vi "MeasLeakRate_20.vi"() -> ()   [LabVIEW 2011]
panel:
  out "angle (°)":dbl
  out "Status":string
  out "error out":errorcluster
  out "fit":cluster{"element":dbl, "Value":dbl}[](array[cluster])
  out "T-T0,P":cluster{"element":dbl, "element":dbl}[](array[cluster])
  out "t0":dbl format="%#_8f"
  out "XY Graph":T1(graph)
  out "S00":i32
  out "S20":dbl
  out "S11":dbl
  out "S10":dbl
  out "S01":dbl
  out "T,P":cluster{"element":dbl, "element":dbl}[](array[cluster])
  out "dPdt":dbl
  out "P0":dbl
  out "average P (Torr)":string
  in  "Control Valve Local":bool
  in  "Exhaust Close":bool
  in  "Exhaust Open":bool
  in  "Control Close":bool
  in  "Control Open":bool
  in  "reset":bool
  in  "# points to watch":i32=60
  out "leak rate (torr/min)":string
  out "P":dbl
  out "first":bool=TRUE
  in  "interval (s)":dbl=0.5
  in  "stop":bool
  out "P(torr)":string
  # "Pressure control valve:"
  # "Exahaust valve:"
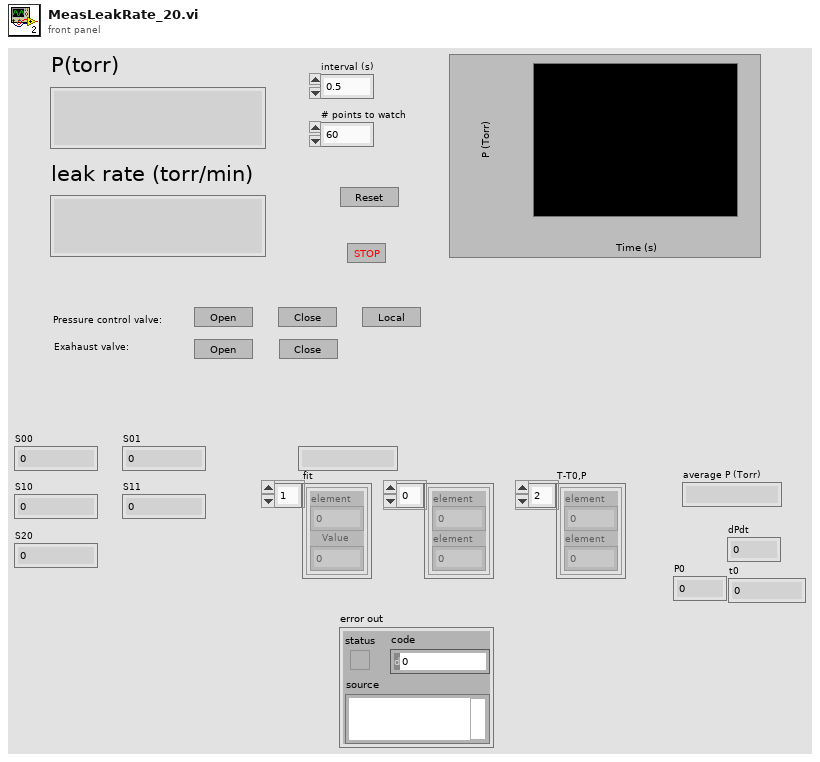
[diagram p1: front panel]
types:
  T1 = cluster{"Value":cluster{"element":dbl, "element":dbl}[]}[]
  T2 = cluster{"Value":cluster{"element":dbl, "Value":dbl}[]}[]
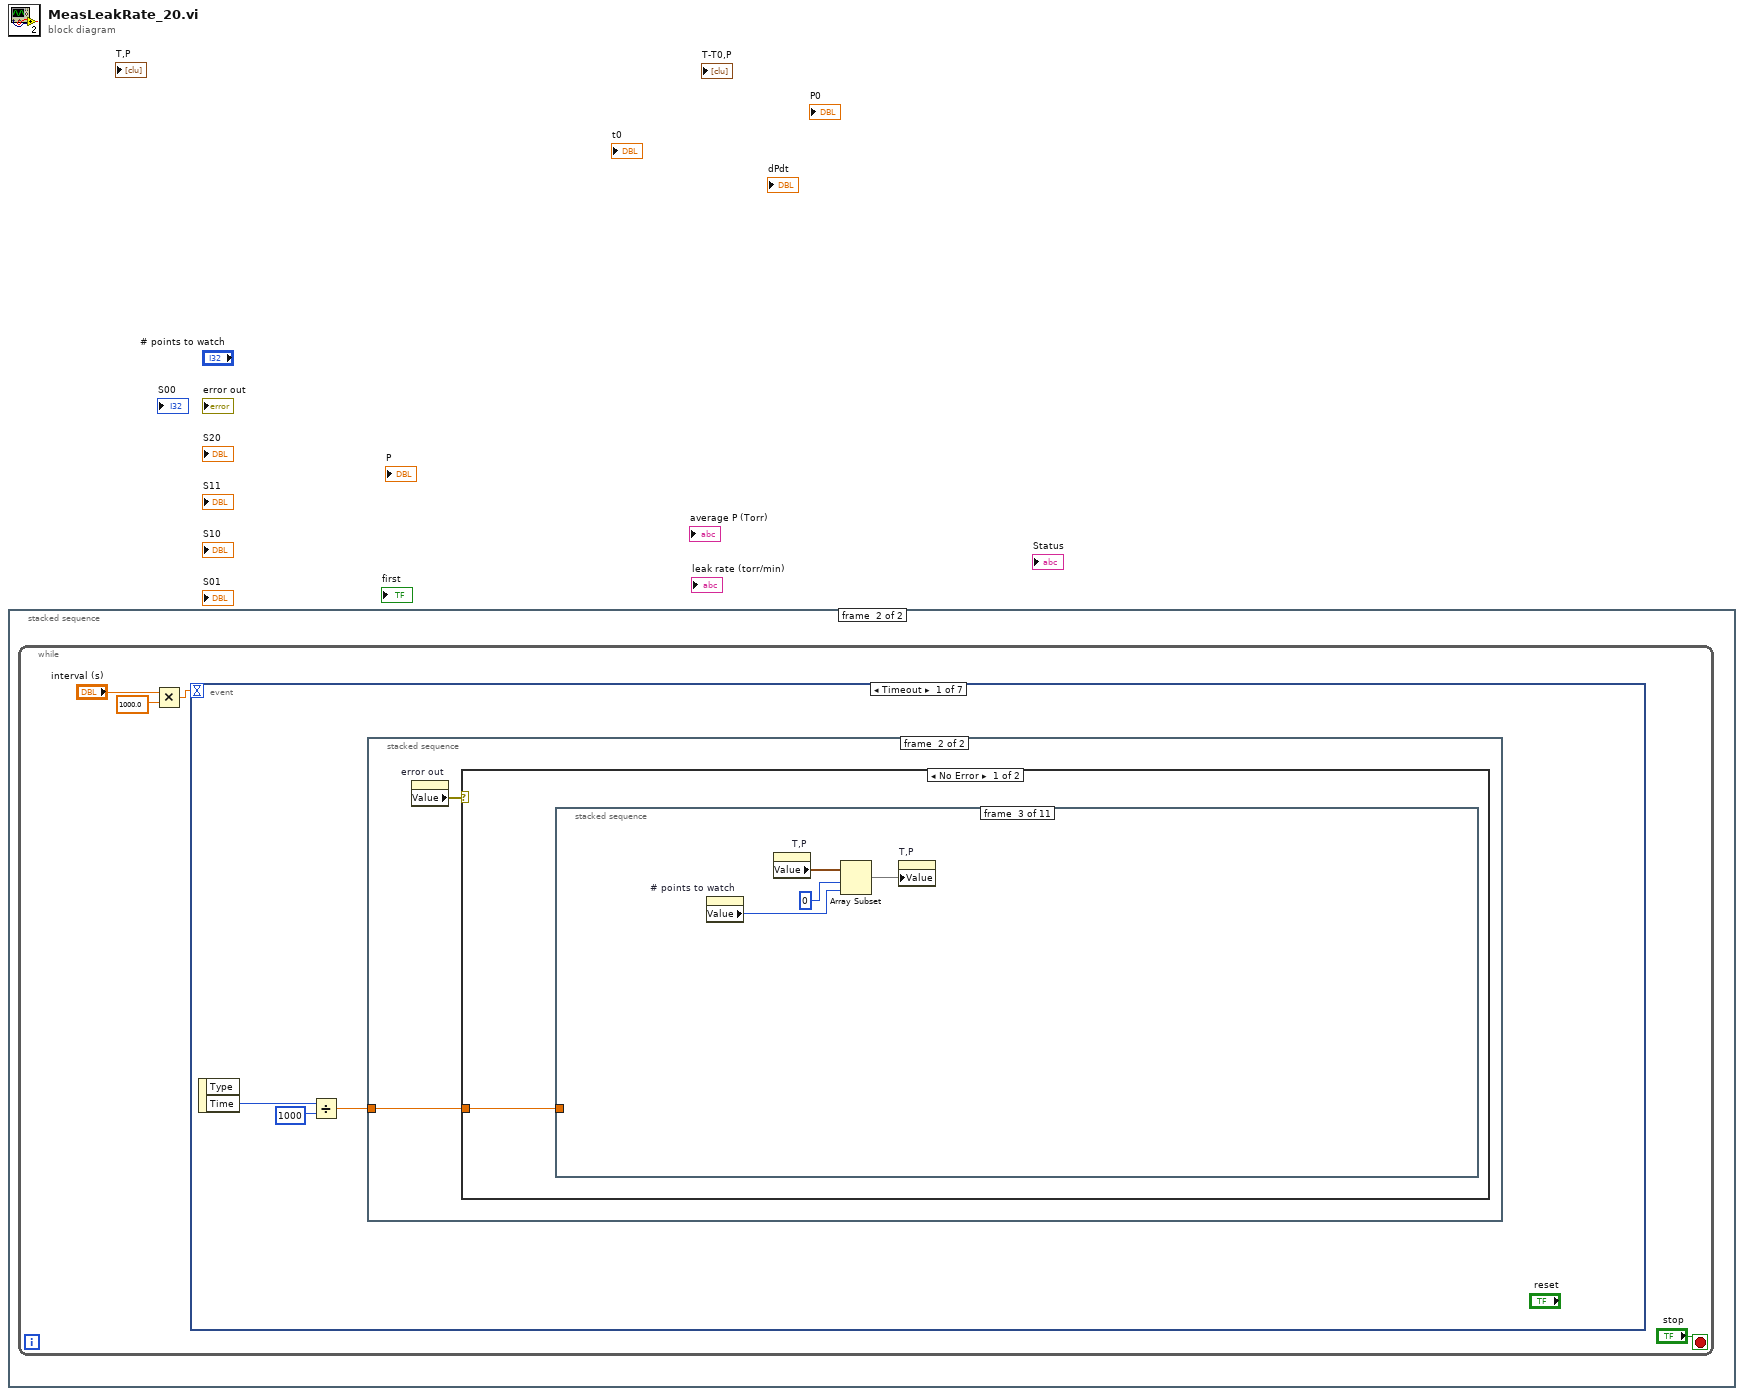
[diagram p0: block diagram]
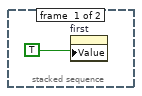
[diagram p2: hidden frame]
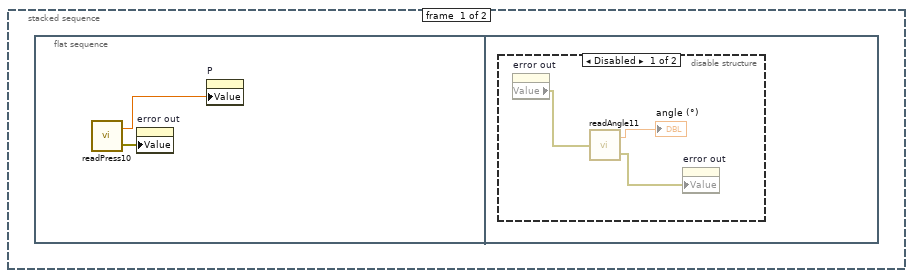
[diagram p3: hidden frame]
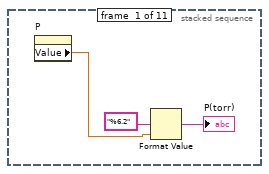
[diagram p5: hidden frame]
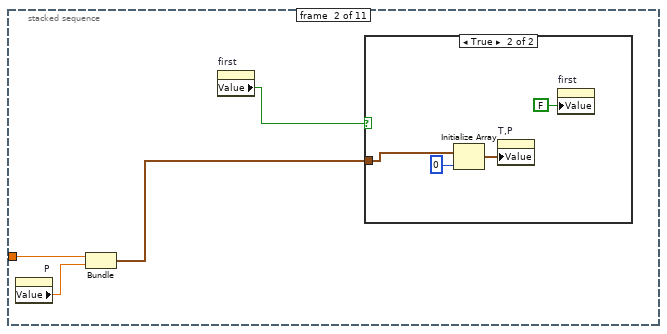
[diagram p6: hidden frame]
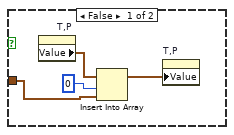
[diagram p7: hidden frame]
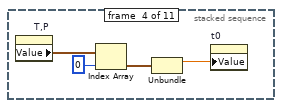
[diagram p8: hidden frame]
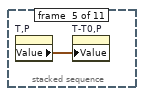
[diagram p9: hidden frame]
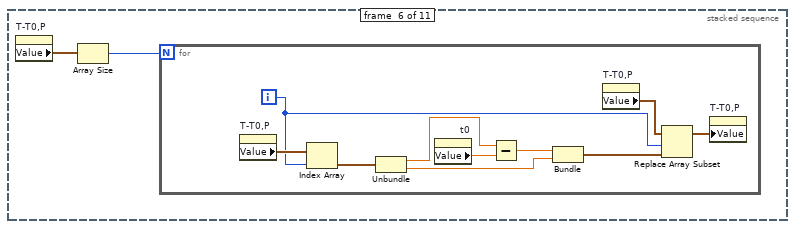
[diagram p10: hidden frame]
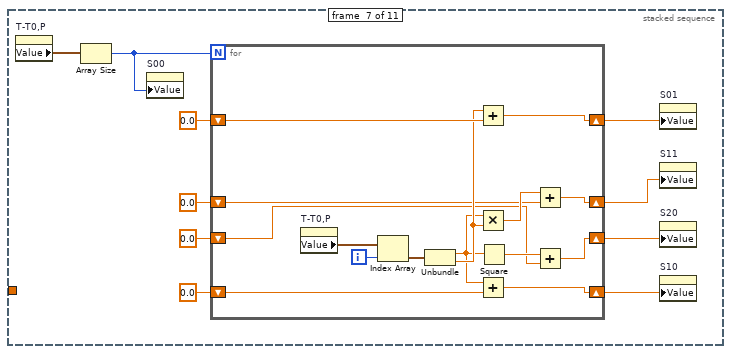
[diagram p11: hidden frame]
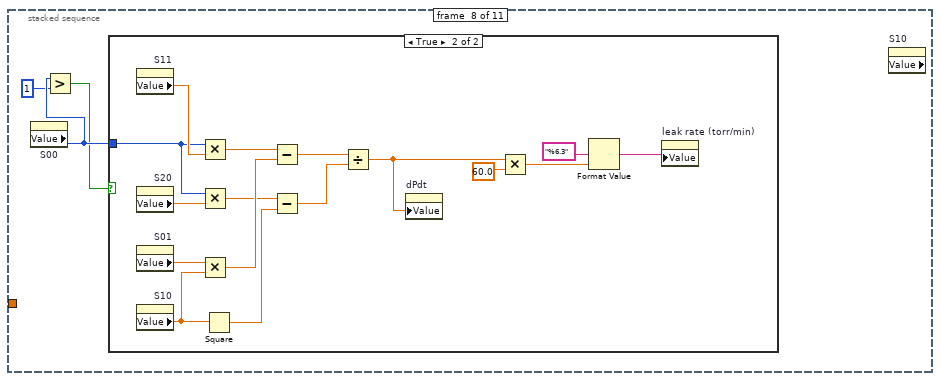
[diagram p12: hidden frame]
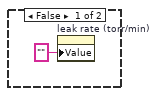
[diagram p13: hidden frame]
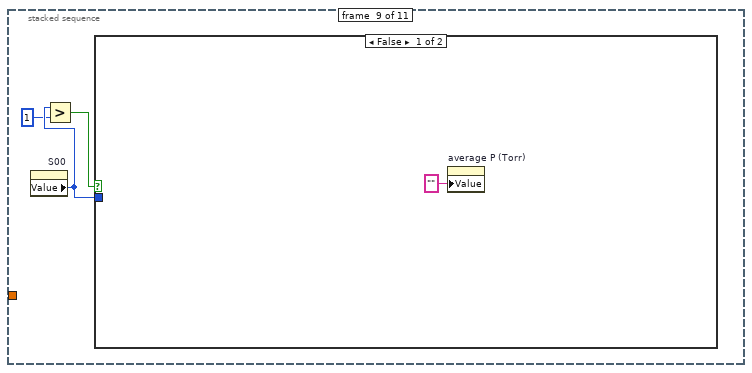
[diagram p14: hidden frame]
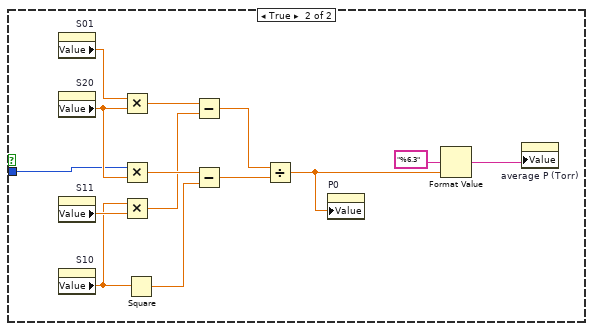
[diagram p15: hidden frame]
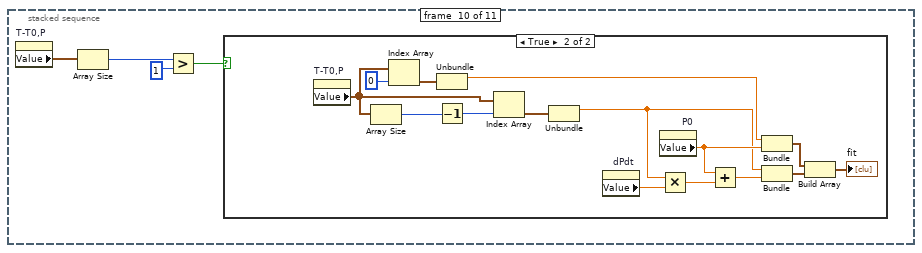
[diagram p16: hidden frame]
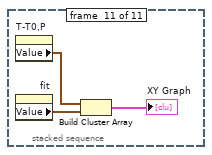
[diagram p18: hidden frame]
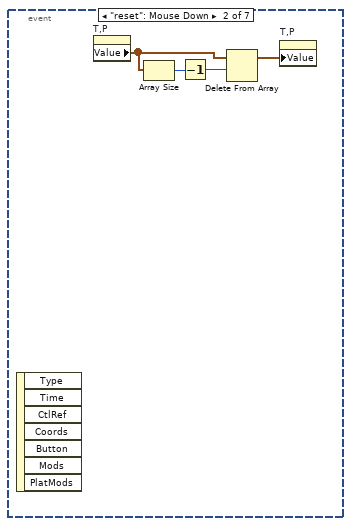
[diagram p20: hidden frame]
diagram:
  n1 = stacked-sequence {
    frame #0 {
      n2 = property on="first" class="Bool (strict)"("Value"=TRUE ("first")) -> ()  [unwired: 2 in, 2 out]
    }
    frame #1 {
      n3 = while {
        stop <- "stop" stop-if-true
        n4 = Multiply(x="interval (s)", y=1000.0) -> (x*y=w3:dbl)
        n5 = event shown="[0] Timeout" {
          selector: _ -> [_ _ _ _ _ _ _]
          dyn-events: _ -> [_ _ _ _ _ _ _]
          timeout: w3 -> [_ _ _ _ _ _ _]
          event Timeout {
            n6 = event-data() -> ("Time"=w8:u32)  [unwired: 1 in, 1 out]
            n7 = Divide(x=w8, y=u32 1000) -> (x/y=w6:dbl)
            n8 = stacked-sequence {
              tunnel: w6 -> [_ w14]
              frame #0 {
                n9 = flat-sequence {
                  frame #0 {
                    n10 = call "readPress10.vi"() -> ("P"=w10:dbl, "error out"=w9:errorcluster)  [unwired: 1 in]
                    n11 = property on="error out" class="Clust (strict)"("Value"=w9) -> ()  [unwired: 2 in, 2 out]
                    n12 = property on="P" class="DigNum (strict)"("Value"=w10) -> ()  [unwired: 2 in, 2 out]
                  }
                  frame #1 {
                    n13 = disable-structure shown="Disabled" {
                      frame Disabled {
                        n14 = property on="error out" class="Clust (strict)"() -> ("Value"=w12:errorcluster)  [unwired: 2 in, 2 out]
                        n15 = call "readAngle11.vi"("error in"=w12) -> ("angle"=→"angle (°)":dbl, "error out"=w11:errorcluster)
                        n16 = property on="error out" class="Clust (strict)"("Value"=w11) -> ()  [unwired: 2 in, 2 out]
                      }
                      frame Enabled {
                      }
                    }
                  }
                }
              }
              frame #1 {
                n17 = property on="error out" class="Clust (strict)"() -> ("Value"=w15:errorcluster)  [unwired: 2 in, 2 out]
                n18 = case shown="No Error" w15 {
                  tunnel: w14 -> [w16 _]
                  frame No Error {
                    n19 = stacked-sequence {
                      tunnel: w16 -> [_ w22 _ _ _ _ _ _ _ _ _]
                      frame #0 {
                        n20 = property on="P" class="DigNum (strict)"() -> ("Value"=w17:dbl)  [unwired: 2 in, 2 out]
                        n21 = Format Value(format string="%6.2", value (0)=w17) -> (output string=→"P(torr)":string)  [unwired: 1 in]
                      }
                      frame #1 {
                        n22 = property on="P" class="DigNum (strict)"() -> ("Value"=w23:dbl)  [unwired: 2 in, 2 out]
                        n23 = Bundle(w22, "Value"=w23) -> (w21:cluster{dbl, "Value":dbl})  [unwired: 1 in]
                        n24 = property on="first" class="Bool (strict)"() -> ("Value"=w20:bool)  [unwired: 2 in, 2 out]
                        n25 = case shown="True" w20 {
                          tunnel: w21 -> [w24 w29]
                          frame False {
                            n26 = property on="T,P" class="Arr (strict)"() -> ("Value"=w25:cluster{"element":dbl, "element":dbl}[])  [unwired: 2 in, 2 out]
                            n27 = Insert Into Array(array=w25, index=0, new element=w24) -> (w27:cluster{"element":dbl, "element":dbl}[])
                            n28 = property on="T,P" class="Arr (strict)"("Value"=w27) -> ()  [unwired: 2 in, 2 out]
                          }
                          frame True {
                            n29 = Initialize Array(w29, 0 ("dimension size")) -> (w30:cluster{dbl, "Value":dbl}[])
                            n30 = property on="T,P" class="Arr (strict)"("Value"=w30) -> ()  [unwired: 2 in, 2 out]
                            n31 = property on="first" class="Bool (strict)"("Value"=FALSE ("first")) -> ()  [unwired: 2 in, 2 out]
                          }
                        }
                      }
                      frame #2 {
                        n32 = property on="# points to watch" class="DigNum (strict)"() -> ("Value"=w33:i32)  [unwired: 2 in, 2 out]
                        n33 = property on="T,P" class="Arr (strict)"() -> ("Value"=w34:cluster{"element":dbl, "element":dbl}[])  [unwired: 2 in, 2 out]
                        n34 = Array Subset(array=w34, index=0, length=w33) -> (w32:cluster{"element":dbl, "element":dbl}[])
                        n35 = property on="T,P" class="Arr (strict)"("Value"=w32) -> ()  [unwired: 2 in, 2 out]
                      }
                      frame #3 {
                        n36 = property on="T,P" class="Arr (strict)"() -> ("Value"=w39:cluster{"element":dbl, "element":dbl}[])  [unwired: 2 in, 2 out]
                        n37 = Index Array(array=w39, index=0) -> (element=w37:cluster{"element":dbl, "element":dbl})
                        n38 = Unbundle(w37) -> ("element"=w36:dbl)  [unwired: 1 out]
                        n39 = property on="t0" class="DigNum (strict)"("Value"=w36) -> ()  [unwired: 2 in, 2 out]
                      }
                      frame #4 {
                        n40 = property on="T,P" class="Arr (strict)"() -> ("Value"=w40:cluster{"element":dbl, "element":dbl}[])  [unwired: 2 in, 2 out]
                        n41 = property on="T-T0,P" class="Arr (strict)"("Value"=w40) -> ()  [unwired: 2 in, 2 out]
                      }
                      frame #5 {
                        n42 = property on="T-T0,P" class="Arr (strict)"() -> ("Value"=w42:cluster{"element":dbl, "element":dbl}[])  [unwired: 2 in, 2 out]
                        n43 = Array Size(array=w42) -> (size(s)=w41:i32)
                        n44 = for {
                          N: w41 -> [_]
                          i -> [w43]
                          n45 = property on="T-T0,P" class="Arr (strict)"() -> ("Value"=w47:cluster{"element":dbl, "element":dbl}[])  [unwired: 2 in, 2 out]
                          n46 = Index Array(array=w47, index=w43) -> (element=w52:cluster{"element":dbl, "element":dbl})
                          n47 = Unbundle(w52) -> ("element"=w51:dbl, "element"=w48:dbl)
                          n48 = property on="t0" class="DigNum (strict)"() -> ("Value"=w50:dbl)  [unwired: 2 in, 2 out]
                          n49 = Subtract(x=w51, y=w50) -> (x-y=w49:dbl)
                          n50 = Bundle(w49, "element"=w48) -> (w46:cluster{dbl, "element":dbl})  [unwired: 1 in]
                          n51 = property on="T-T0,P" class="Arr (strict)"() -> ("Value"=w45:cluster{"element":dbl, "element":dbl}[])  [unwired: 2 in, 2 out]
                          n52 = Replace Array Subset(array=w45, new element=w46, index=w43) -> (w44:cluster{"element":dbl, "element":dbl}[])
                          n53 = property on="T-T0,P" class="Arr (strict)"("Value"=w44) -> ()  [unwired: 2 in, 2 out]
                        }
                      }
                      frame #6 {
                        n54 = property on="T-T0,P" class="Arr (strict)"() -> ("Value"=w53:cluster{"element":dbl, "element":dbl}[])  [unwired: 2 in, 2 out]
                        n55 = Array Size(array=w53) -> (size(s)=w57:i32)
                        n56 = property on="S00" class="DigNum (strict)"("Value"=w57) -> ()  [unwired: 2 in, 2 out]
                        n57 = for {
                          N: w57 -> [_]
                          shift-right: [w75] -> w56
                          shift-left: 0.0 -> [w77]
                          shift-right: [w74] -> w60
                          shift-left: 0.0 -> [w73]
                          shift-right: [w70] -> w55
                          shift-left: 0.0 -> [w69]
                          shift-right: [w66] -> w54
                          shift-left: 0.0 -> [w65]
                          i -> [w64]
                          n58 = property on="T-T0,P" class="Arr (strict)"() -> ("Value"=w63:cluster{"element":dbl, "element":dbl}[])  [unwired: 2 in, 2 out]
                          n59 = Index Array(array=w63, index=w64) -> (element=w76:cluster{"element":dbl, "element":dbl})
                          n60 = Unbundle(w76) -> ("element"=w68:dbl, "element"=w72:dbl)
                          n61 = Add(x=w72, y=w73) -> (x+y=w74:dbl)
                          n62 = Multiply(x=w68, y=w72) -> (x*y=w71:dbl)
                          n63 = Add(x=w68, y=w77) -> (x+y=w75:dbl)
                          n64 = Square(x=w68) -> (x^2=w67:dbl)
                          n65 = Add(x=w71, y=w69) -> (x+y=w70:dbl)
                          n66 = Add(x=w67, y=w65) -> (x+y=w66:dbl)
                        }
                        n67 = property on="S01" class="DigNum (strict)"("Value"=w60) -> ()  [unwired: 2 in, 2 out]
                        n68 = property on="S11" class="DigNum (strict)"("Value"=w55) -> ()  [unwired: 2 in, 2 out]
                        n69 = property on="S20" class="DigNum (strict)"("Value"=w54) -> ()  [unwired: 2 in, 2 out]
                        n70 = property on="S10" class="DigNum (strict)"("Value"=w56) -> ()  [unwired: 2 in, 2 out]
                      }
                      frame #7 {
                        n71 = property on="S00" class="DigNum (strict)"() -> ("Value"=w80:i32)  [unwired: 2 in, 2 out]
                        n72 = Greater?(x=w80, y=1) -> (0:w78:bool)
                        n73 = case shown="True" w78 {
                          tunnel: w80 -> [_ w85]
                          frame False {
                            n74 = property on="leak rate (torr/min)" class="Str"("Value"="" ("leak rate (Torr/min)")) -> ()  [unwired: 2 in, 2 out]
                          }
                          frame True {
                            n75 = property on="S11" class="DigNum (strict)"() -> ("Value"=w87:dbl)  [unwired: 2 in, 2 out]
                            n76 = property on="S20" class="DigNum (strict)"() -> ("Value"=w86:dbl)  [unwired: 2 in, 2 out]
                            n77 = property on="S01" class="DigNum (strict)"() -> ("Value"=w84:dbl)  [unwired: 2 in, 2 out]
                            n78 = property on="S10" class="DigNum (strict)"() -> ("Value"=w88:dbl)  [unwired: 2 in, 2 out]
                            n79 = Multiply(x=w85, y=w87) -> (x*y=w97:dbl)
                            n80 = Multiply(x=w85, y=w86) -> (x*y=w95:dbl)
                            n81 = Multiply(x=w84, y=w88) -> (x*y=w96:dbl)
                            n82 = Square(x=w88) -> (x^2=w94:dbl)
                            n83 = Subtract(x=w97, y=w96) -> (x-y=w93:dbl)
                            n84 = Subtract(x=w95, y=w94) -> (x-y=w92:dbl)
                            n85 = Divide(x=w93, y=w92) -> (x/y=w83:dbl)
                            n86 = property on="dPdt" class="DigNum (strict)"("Value"=w83) -> ()  [unwired: 2 in, 2 out]
                            n87 = Multiply(x=w83, y=60.0) -> (x*y=w89:dbl)
                            n88 = Format Value(format string="%6.3", value (0)=w89) -> (output string=w82:string)  [unwired: 1 in]
                            n89 = property on="leak rate (torr/min)" class="Str"("Value"=w82) -> ()  [unwired: 2 in, 2 out]
                          }
                        }
                        n90 = property on="S10" class="DigNum (strict)" props=["Value"]() -> ()  [unwired: 2 in, 3 out]
                      }
                      frame #8 {
                        n91 = property on="S00" class="DigNum (strict)"() -> ("Value"=w100:i32)  [unwired: 2 in, 2 out]
                        n92 = Greater?(x=w100, y=1) -> (0:w98:bool)
                        n93 = case shown="False" w98 {
                          tunnel: w100 -> [_ w103]
                          frame False {
                            n94 = property on="average P (Torr)" class="Str"("Value"="" ("average P (Torr)")) -> ()  [unwired: 2 in, 2 out]
                          }
                          frame True {
                            n95 = property on="S01" class="DigNum (strict)"() -> ("Value"=w115:dbl)  [unwired: 2 in, 2 out]
                            n96 = property on="S20" class="DigNum (strict)"() -> ("Value"=w112:dbl)  [unwired: 2 in, 2 out]
                            n97 = property on="S11" class="DigNum (strict)"() -> ("Value"=w114:dbl)  [unwired: 2 in, 2 out]
                            n98 = property on="S10" class="DigNum (strict)"() -> ("Value"=w113:dbl)  [unwired: 2 in, 2 out]
                            n99 = Multiply(x=w115, y=w112) -> (x*y=w105:dbl)
                            n100 = Multiply(x=w103, y=w112) -> (x*y=w108:dbl)
                            n101 = Multiply(x=w113, y=w114) -> (x*y=w104:dbl)
                            n102 = Square(x=w113) -> (x^2=w107:dbl)
                            n103 = Subtract(x=w105, y=w104) -> (x-y=w111:dbl)
                            n104 = Subtract(x=w108, y=w107) -> (x-y=w106:dbl)
                            n105 = Divide(x=w111, y=w106) -> (x/y=w109:dbl)
                            n106 = property on="P0" class="DigNum (strict)"("Value"=w109) -> ()  [unwired: 2 in, 2 out]
                            n107 = Format Value(format string="%6.3", value (0)=w109) -> (output string=w102:string)  [unwired: 1 in]
                            n108 = property on="average P (Torr)" class="Str"("Value"=w102) -> ()  [unwired: 2 in, 2 out]
                          }
                        }
                      }
                      frame #9 {
                        n109 = property on="T-T0,P" class="Arr (strict)"() -> ("Value"=w119:cluster{"element":dbl, "element":dbl}[])  [unwired: 2 in, 2 out]
                        n110 = Array Size(array=w119) -> (size(s)=w118:i32)
                        n111 = Greater?(x=w118, y=1) -> (0:w116:bool)
                        n112 = case shown="True" w116 {
                          frame False {
                          }
                          frame True {
                            n113 = property on="T-T0,P" class="Arr (strict)"() -> ("Value"=w123:cluster{"element":dbl, "element":dbl}[])  [unwired: 2 in, 2 out]
                            n114 = Array Size(array=w123) -> (size(s)=w133:i32)
                            n115 = Index Array(array=w123, index=0) -> (element=w131:cluster{"element":dbl, "element":dbl})
                            n116 = Unbundle(w131) -> ("element"=w126:dbl)  [unwired: 1 out]
                            n117 = Decrement(x=w133) -> (x-1=w132:i32)
                            n118 = Index Array(array=w123, index=w132) -> (element=w130:cluster{"element":dbl, "element":dbl})
                            n119 = Unbundle(w130) -> ("element"=w124:dbl)  [unwired: 1 out]
                            n120 = property on="dPdt" class="DigNum (strict)"() -> ("Value"=w129:dbl)  [unwired: 2 in, 2 out]
                            n121 = property on="P0" class="DigNum (strict)"() -> ("Value"=w127:dbl)  [unwired: 2 in, 2 out]
                            n122 = Multiply(x=w124, y=w129) -> (x*y=w128:dbl)
                            n123 = Add(x=w127, y=w128) -> (x+y=w125:dbl)
                            n124 = Bundle("element"=w126, "Value"=w127) -> (w122:cluster{"element":dbl, "Value":dbl})  [unwired: 1 in]
                            n125 = Bundle("element"=w124, w125) -> (w121:cluster{"element":dbl, dbl})  [unwired: 1 in]
                            n126 = Build Array(w122, w121) -> (→"fit":cluster{"element":dbl, "Value":dbl}[])
                          }
                        }
                      }
                      frame #10 {
                        n127 = property on="T-T0,P" class="Arr (strict)"() -> ("Value"=w137:cluster{"element":dbl, "element":dbl}[])  [unwired: 2 in, 2 out]
                        n128 = property on="fit" class="Arr (strict)"() -> ("Value"=w135:cluster{"element":dbl, "Value":dbl}[])  [unwired: 2 in, 2 out]
                        n129 = Build Cluster Array(w137, w135) -> (→"XY Graph":T2)
                      }
                    }
                  }
                  frame Error {
                  }
                }
              }
            }
          }
          event "reset": Mouse Down {
            n130 = event-data() -> ()  [unwired: 1 in, 7 out]
            n131 = property on="T,P" class="Arr (strict)"() -> ("Value"=w139:cluster{"element":dbl, "element":dbl}[])  [unwired: 2 in, 2 out]
            n132 = Array Size(array=w139) -> (size(s)=w141:i32)
            n133 = Decrement(x=w141) -> (x-1=w140:i32)
            n134 = Delete From Array(array=w139, length=w140) -> (array with subset deleted=w138:cluster{"element":dbl, "element":dbl}[])  [unwired: 1 in, 1 out]
            n135 = property on="T,P" class="Arr (strict)"("Value"=w138) -> ()  [unwired: 2 in, 2 out]
          }
          event "Control Open": Mouse Up {
            n136 = event-data() -> ()  [unwired: 1 in, 7 out]
            n137 = case shown="True" "Control Open" {
              frame False {
              }
              frame True {
                n138 = stacked-sequence {
                  frame #0 {
                    n139 = call "WriteAdaptorr03.vi"("string to write"="O") -> ()  [unwired: 1 in, 1 out]
                  }
                  frame #1 {
                    n140 = Wait (ms)(milliseconds to wait=u32 1000) -> ()  [unwired: 1 out]
                    n141 = while {
                      stop <- w146 stop-if-true
                      n142 = call "readStatus_00.vi"() -> ("Status"=w145:string, "error out"=w147:errorcluster)  [unwired: 1 in, 1 out]
                      n143 = property on="Status" class="Str"("Value"=w145) -> ()  [unwired: 2 in, 2 out]
                      n144 = property on="error out" class="Clust (strict)"("Value"=w147) -> ()  [unwired: 2 in, 2 out]
                      n145 = case shown="Default" w145 {
                        tunnel: [FALSE TRUE] -> w146
                        frame Default {
                        }
                        frame "Open" {
                        }
                      }
                    }
                  }
                  frame #2 {
                    n146 = property on="Control Open" class="Bool (strict)"("Value"=FALSE) -> ()  [unwired: 2 in, 2 out]
                  }
                  frame #3 {
                    n147 = call "WriteAdaptorr03.vi"("string to write"="D5") -> ()  [unwired: 1 in, 1 out]
                  }
                }
              }
            }
          }
          event "Control Close": Mouse Up {
            n148 = event-data() -> ()  [unwired: 1 in, 7 out]
            n149 = case shown="True" "Control Close" {
              frame False {
              }
              frame True {
                n150 = stacked-sequence {
                  frame #0 {
                    n151 = call "WriteAdaptorr03.vi"("string to write"="C") -> ()  [unwired: 1 in, 1 out]
                  }
                  frame #1 {
                    n152 = while {
                      stop <- w156 stop-if-true
                      n153 = call "readStatus_00.vi"() -> ("Status"=w154:string, "error out"=w155:errorcluster)  [unwired: 1 in, 1 out]
                      n154 = property on="Status" class="Str"("Value"=w154) -> ()  [unwired: 2 in, 2 out]
                      n155 = property on="error out" class="Clust (strict)"("Value"=w155) -> ()  [unwired: 2 in, 2 out]
                      n156 = case shown="\"Closed\"" w154 {
                        tunnel: [FALSE TRUE] -> w156
                        frame Default {
                        }
                        frame "Closed" {
                        }
                      }
                    }
                  }
                  frame #2 {
                    n157 = property on="Control Close" class="Bool (strict)"("Value"=FALSE) -> ()  [unwired: 2 in, 2 out]
                  }
                  frame #3 {
                    n158 = call "WriteAdaptorr03.vi"("string to write"="D5") -> ()  [unwired: 1 in, 1 out]
                  }
                }
              }
            }
          }
          event "Exhaust Open": Mouse Up {
            n159 = event-data() -> ()  [unwired: 1 in, 7 out]
            n160 = case shown="True" "Exhaust Open" {
              frame False {
              }
              frame True {
                n161 = call "set_vacuum.vi"("Remote"=TRUE ("Vac Remote"), "Atm"=FALSE ("Atm Exhaust"), "Vac Exhaust"=TRUE) -> ()
              }
            }
          }
          event "Exhaust Close": Mouse Up {
            n162 = event-data() -> ()  [unwired: 1 in, 7 out]
            n163 = case shown="True" "Exhaust Close" {
              frame False {
              }
              frame True {
                n164 = call "set_vacuum.vi"("Remote"=TRUE ("Vac Remote"), "Atm"=FALSE ("Atm Exhaust"), "Vac Exhaust"=FALSE) -> ()
              }
            }
          }
          event "Control Valve Local": Mouse Up {
            n165 = event-data() -> ()  [unwired: 1 in, 7 out]
            n166 = case shown="True" "Control Valve Local" {
              frame False {
              }
              frame True {
                n167 = call "WriteAdaptorr03.vi"("string to write"="D5") -> ()  [unwired: 1 in, 1 out]
              }
            }
          }
        }
      }
    }
  }
